vi "IO Template.vi"(2 "Enum":enum16{"Start", "Run", "End"}(ring)) -> ()   [LabVIEW 2013]
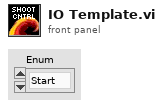
[diagram p1: front panel]
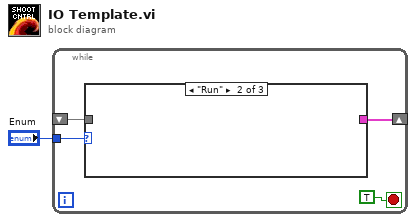
[diagram p0: block diagram]
diagram:
  n1 = while {
    tunnel: "Enum" -> [w4]
    shift-right: [w2] -> _
    shift-left: _ -> [w3]
    stop <- TRUE stop-if-true
    n2 = case shown="\"Run\"" w4 {
      tunnel: w3 -> [_ _ _]
      tunnel: [_ _ _] -> w2
      frame "Start", Default {
      }
      frame "Run" {
      }
      frame "End" {
      }
    }
  }
